vi "查找替换数组元素(2D TimeStamp).vi"(7 "开始索引（0）":i32, 8 "error in (no error)":errorcluster caption="错误输入（无错误）", 9 "替换值":timestamp, 10 "查找元素":timestamp, 11 "输入数组":timestamp[][](array[timestamp])) -> (0 "error out":errorcluster caption="错误输出", 2 "匹配元素索引":cluster{"行":i32, "列":i32}[](array[cluster]), 3 "输出数组":timestamp[][](array[timestamp]))   [LabVIEW 2012]
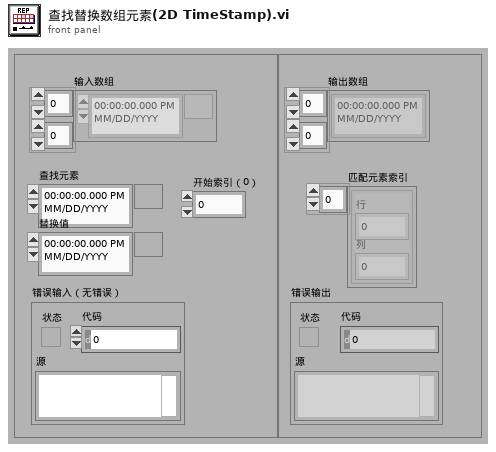
[diagram p1: front panel]
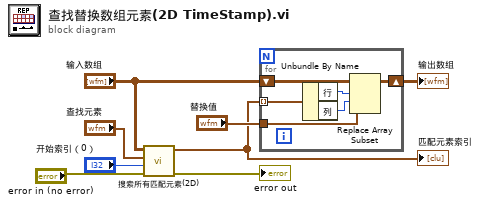
[diagram p0: block diagram]
diagram:
  n1 = call-poly "搜索所有匹配元素(2D).vi"("error in (no error)"="error in (no error)", "开始索引（0）"="开始索引（0）", "元素"="查找元素", "数组"="输入数组") -> ("error out"=→"error out":errorcluster, "匹配元素索引"=w1:cluster{"行":i32, "列":i32}[])  [unwired: 5 in, 1 out]
  "匹配元素索引" <- w1
  n2 = for {
    tunnel: w1 -> [w12] mode=indexing
    shift-right: [w13] -> w3
    shift-left: "输入数组" -> [w14]
    tunnel: "替换值" -> [w9]
    n3 = Unbundle By Name(w12) -> ("行"=w11:i32, "列"=w10:i32)
    n4 = Replace Array Subset(array=w14, new element=w9, index (row)=w11, index (col)=w10) -> (w13:timestamp[][])
  }
  "输出数组" <- w3
